vi "WPI_ADI_IMU_Accumulation_Reset.vi"(3 "AHRS Reset In":T1, 4 "Reset?":bool, 5 "Absolute Angle In":T2) -> (0 "AHRS Reset Out":T1, 2 "Converted Output":T2)   [LabVIEW 2015, in "FRC ADI MXP IMU.lvlib"]
uses:
  FRC ADI MXP IMU.lvlib
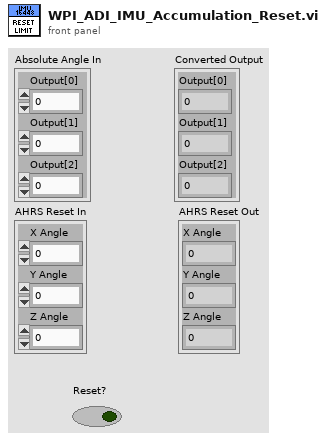
[diagram p1: front panel]
types:
  T1 = cluster{"X Angle":dbl, "Y Angle":dbl, "Z Angle":dbl}
  T2 = cluster{"Output[0]":dbl, "Output[1]":dbl, "Output[2]":dbl}
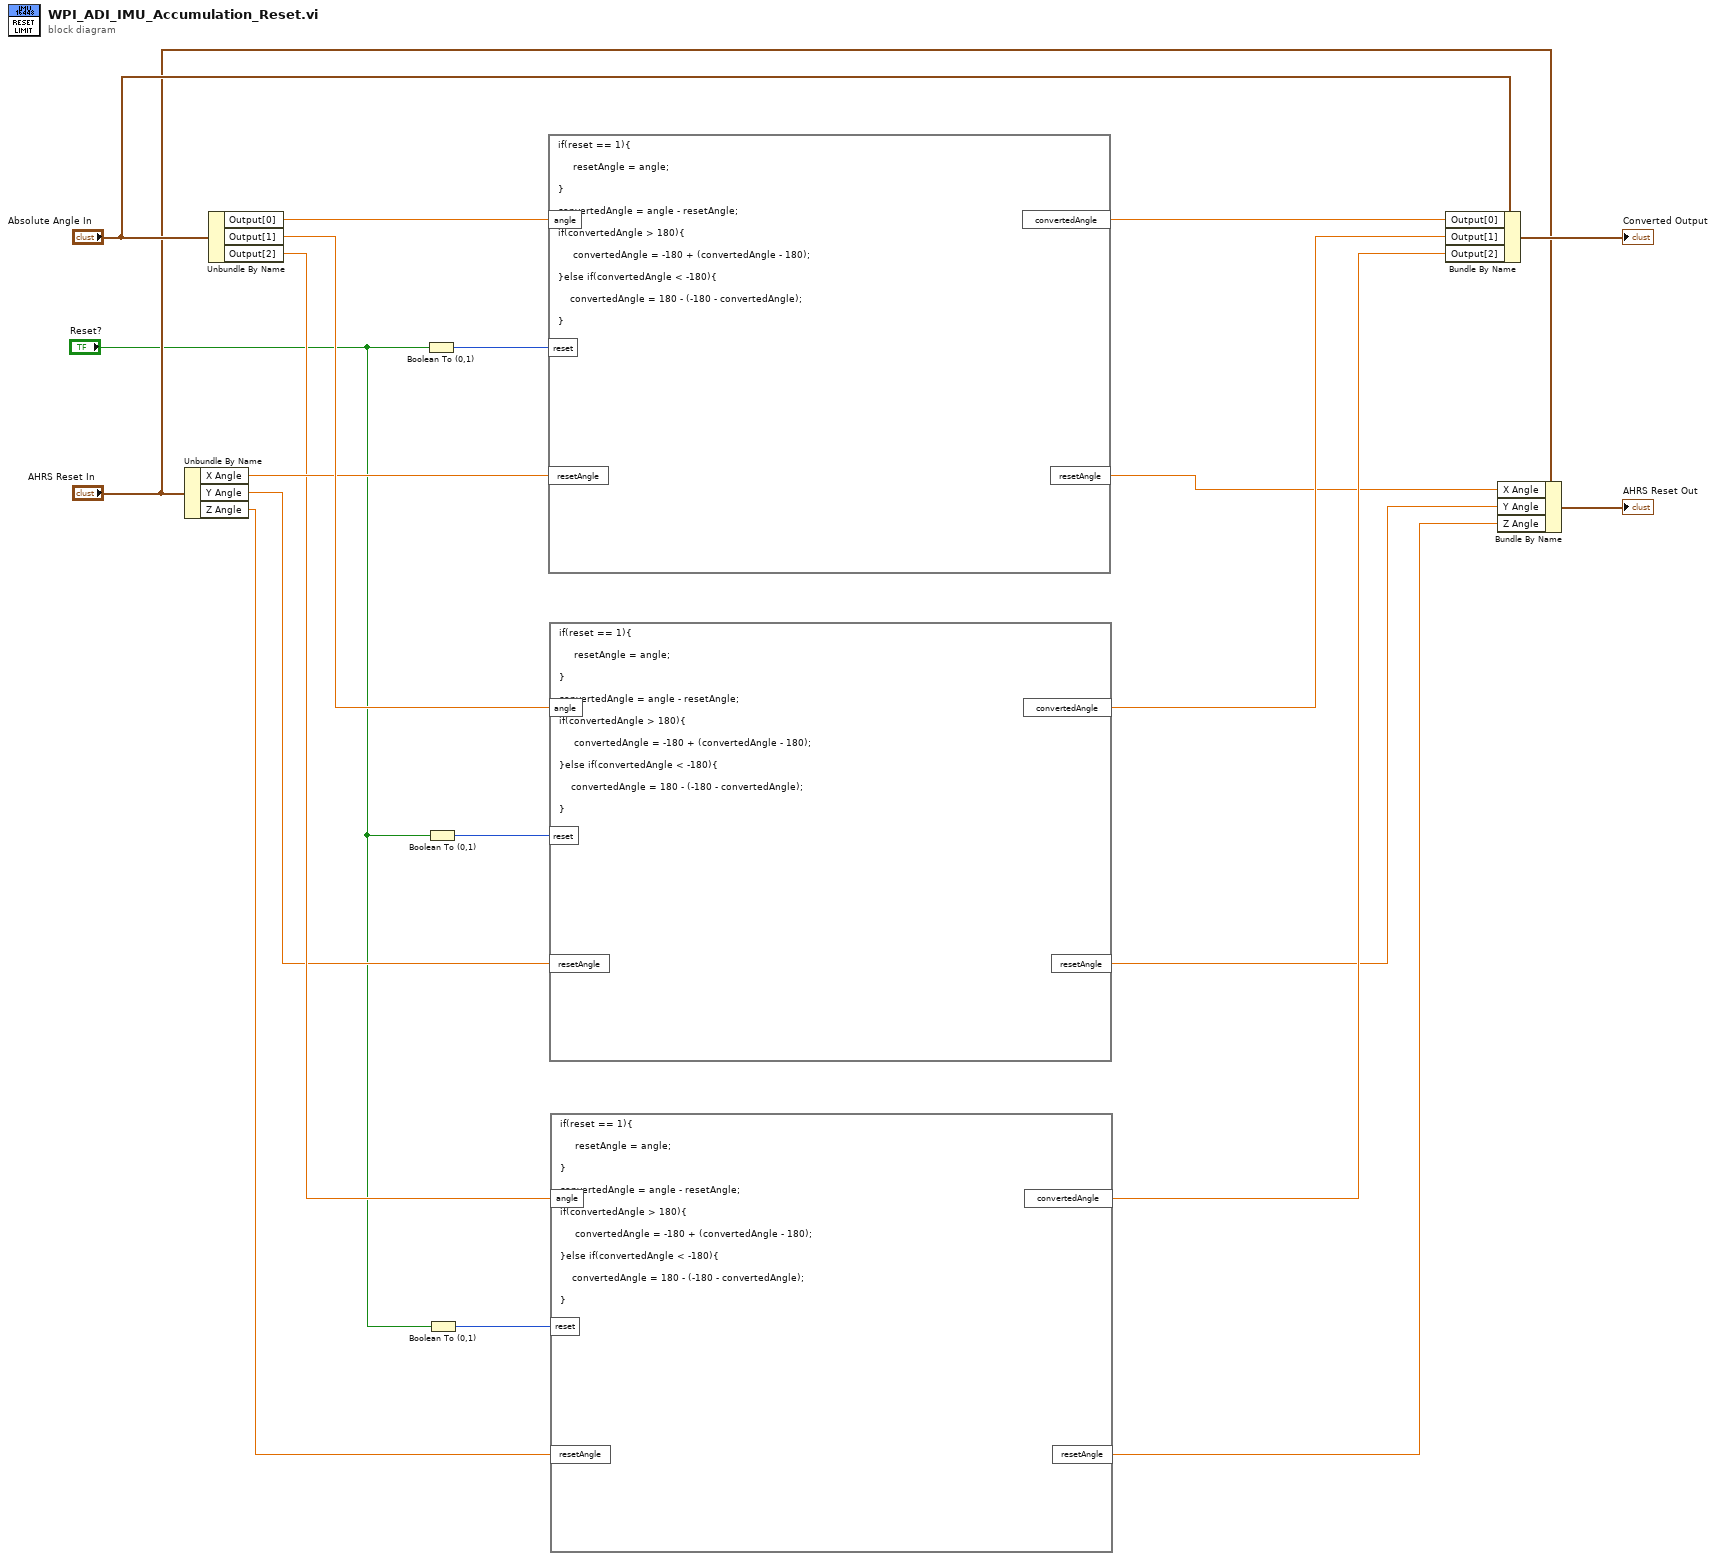
[diagram p0: block diagram]
diagram:
  n1 = Unbundle By Name("AHRS Reset In") -> ("X Angle"=w15:dbl, "Y Angle"=w13:dbl, "Z Angle"=w12:dbl)
  n2 = Unbundle By Name("Absolute Angle In") -> ("Output[0]"=w17:dbl, "Output[1]"=w16:dbl, "Output[2]"=w14:dbl)
  n3 = Boolean To (0,1)(Boolean="Reset?") -> (0, 1=w20:i16)
  n4 = Boolean To (0,1)(Boolean="Reset?") -> (0, 1=w19:i16)
  n5 = Boolean To (0,1)(Boolean="Reset?") -> (0, 1=w18:i16)
  n6 = formula code="if(reset == 1){\n\t\t\t\n\t\t\t  resetAngle = angle;\n\n}\n\t\t\nconvertedAngle = angle - resetAngle;\n\t\t\nif(convertedAngle > 180){\n\t\t\t\n\t\t\t  convertedAngle = -180 + (convertedAngle - 180);\n\t\t\t\n}else if(convertedAngle < -180){\n\t\t\t\n\t\t  convertedAngle = 180 - (-180 - convertedAngle);\n\t\t\t\n}"("angle"=w17, "reset"=w20, "resetAngle"=w15) -> ("convertedAngle"=w9:dbl, "resetAngle"=w4:dbl)
  n7 = formula code="if(reset == 1){\n\t\t\t\n\t\t\t  resetAngle = angle;\n\n}\n\t\t\nconvertedAngle = angle - resetAngle;\n\t\t\nif(convertedAngle > 180){\n\t\t\t\n\t\t\t  convertedAngle = -180 + (convertedAngle - 180);\n\t\t\t\n}else if(convertedAngle < -180){\n\t\t\t\n\t\t  convertedAngle = 180 - (-180 - convertedAngle);\n\t\t\t\n}"("angle"=w16, "reset"=w19, "resetAngle"=w13) -> ("convertedAngle"=w8:dbl, "resetAngle"=w3:dbl)
  n8 = formula code="if(reset == 1){\n\t\t\t\n\t\t\t  resetAngle = angle;\n\n}\n\t\t\nconvertedAngle = angle - resetAngle;\n\t\t\nif(convertedAngle > 180){\n\t\t\t\n\t\t\t  convertedAngle = -180 + (convertedAngle - 180);\n\t\t\t\n}else if(convertedAngle < -180){\n\t\t\t\n\t\t  convertedAngle = 180 - (-180 - convertedAngle);\n\t\t\t\n}"("angle"=w14, "reset"=w18, "resetAngle"=w12) -> ("convertedAngle"=w7:dbl, "resetAngle"=w2:dbl)
  n9 = Bundle By Name(cluster="Absolute Angle In", "Output[0]"=w9, "Output[1]"=w8, "Output[2]"=w7) -> (→"Converted Output":T2)
  n10 = Bundle By Name(cluster="AHRS Reset In", "X Angle"=w4, "Y Angle"=w3, "Z Angle"=w2) -> (→"AHRS Reset Out":T1)
